vi "Configure OVP Core.vi"(6 "enabled (true)":bool=TRUE, 8 "error in (no error)":errorcluster, 9 "limit (0.0 Volts)":dbl[unit] format="%^.2e", 10 "channel name (\"CHANNEL1\")":string="CHANNEL1", 11 "IVI_DCPwr in":refnum<class "IVI_DCPwr.lvclass">) -> (0 "error out":errorcluster, 3 "IVI_DCPwr out":refnum<class "IVI_DCPwr.lvclass">)   [LabVIEW 2015, in "IVI_DCPwr.lvlib" / "IVI_DCPwr.lvclass"]
doc: "This VI configures the power supply's over-voltage protection. You specify the over-voltage limit and the behavior of the power supply when the output voltage is greater than or equal to that value.\n\nWhen the enabled parameter is FALSE, the limit parameter does not affect the instrument's behavior, and the driver ignores the limit parameter."
uses:
  IVI_DCPwr.lvclass
  IVI_DCPwr.lvclass/IVI_DCPwr.ctl
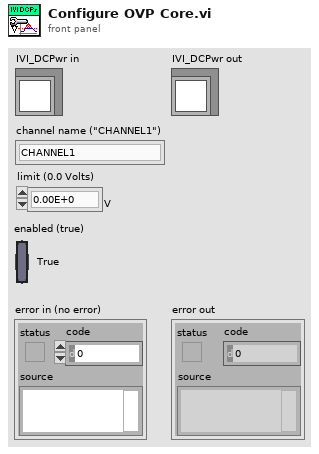
[diagram p1: front panel]
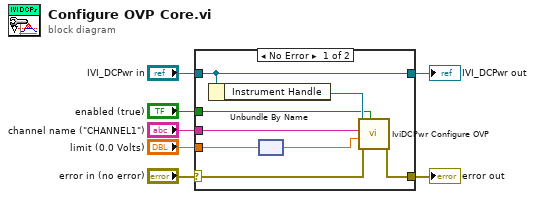
[diagram p0: block diagram]
diagram:
  n1 = case shown="No Error" "error in (no error)" {
    selector: "error in (no error)" -> [w13 w17]
    tunnel: [w12 w17] -> w6
    tunnel: [w15 w16] -> w4
    tunnel: "IVI_DCPwr in" -> [w15 w16]
    tunnel: "channel name (\"CHANNEL1\")" -> [w11 _]
    tunnel: "limit (0.0 Volts)" -> [w10 _]
    tunnel: "enabled (true)" -> [w9 _]
    frame No Error {
      n2 = Unbundle By Name(w15) -> ("Instrument Handle"=w14:refnum<k15>)
      n3 = node(w10) -> (w8:dbl)
      n4 = call <vilib>:"IviDCPwr Configure OVP.vi"("enabled (true)"=w9, "error in (no error)"=w13, "limit (0.0 Volts)"=w8, "channel name (\"CHANNEL1\")"=w11, "instrument handle"=w14) -> ("error out"=w12:errorcluster)  [unwired: 5 in, 1 out]
    }
    frame Error {
    }
  }
  "error out" <- w6
  "IVI_DCPwr out" <- w4
